vi "PH_Cam_BaseClass.get Cam Attribute.vi"(0 "IMAQ1394 Session In":T3, 1 "Cam Number Attribute Name":string, 2 "Attribute Information Array":T2(array[cluster]), 5 "error in (no error)":errorcluster) -> (6 "Current String Value":string, 7 "Attribute writable?":bool, 8 "Current Bool Value":bool, 9 "EnumValues[]":u32[](array[numeric]), 10 "Comment/Attribute Type":string, 11 "EnumStrings[]":string[](array[string]), 12 "Attribute read?":bool, 13 "Description":string, 14 "IMAQ1394 Session Out":T3, 15 "Current Num Value":dbl, 16 "Maximum":dbl, 17 "Minimum":dbl, 18 "Units":string, 19 "error out":errorcluster)   [LabVIEW 2014]
doc: "This VI gets a camera attribute."
uses:
  <vilib>/userdefined/High Color/IMAQdx.ctl
  <vilib>/vision/driver/IMAQdx.llb/IMAQdx Attribute Type.ctl
  <resource>/objmgr/imaqdx.rc
  <vilib>/vision/driver/NI_Vision_Acquisition_Software.lvlib
panel:
  in  "Attribute Type":T1
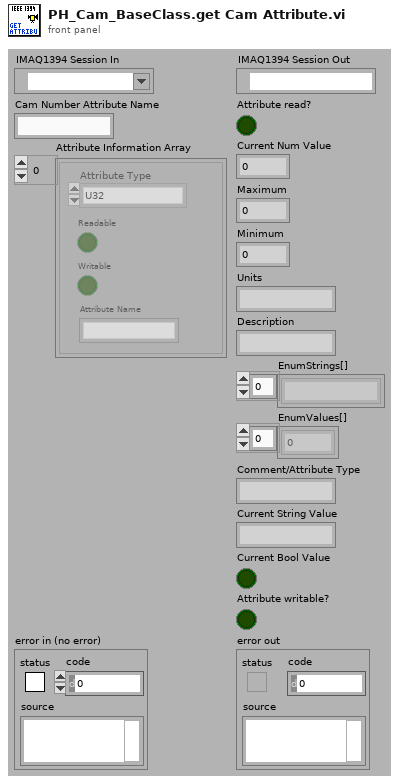
[diagram p1: front panel]
types:
  T1 = typedef "NI_Vision_Acquisition_Software.lvlib/IMAQdx Attribute Type.ctl" = enum32{"U32", "I64", "DBL", "String", "Enum", "Bool", "Command"}
  T2 = cluster{"Attribute Type":T1, "Readable":bool, "Writable":bool, "Attribute Name":string}[]
  T3 = typedef "IMAQdx.ctl" = refnum<k21>
  T4 = cluster{"Attribute Type":T1, "Readable":bool, "Writable":bool, "Attribute Name":string}
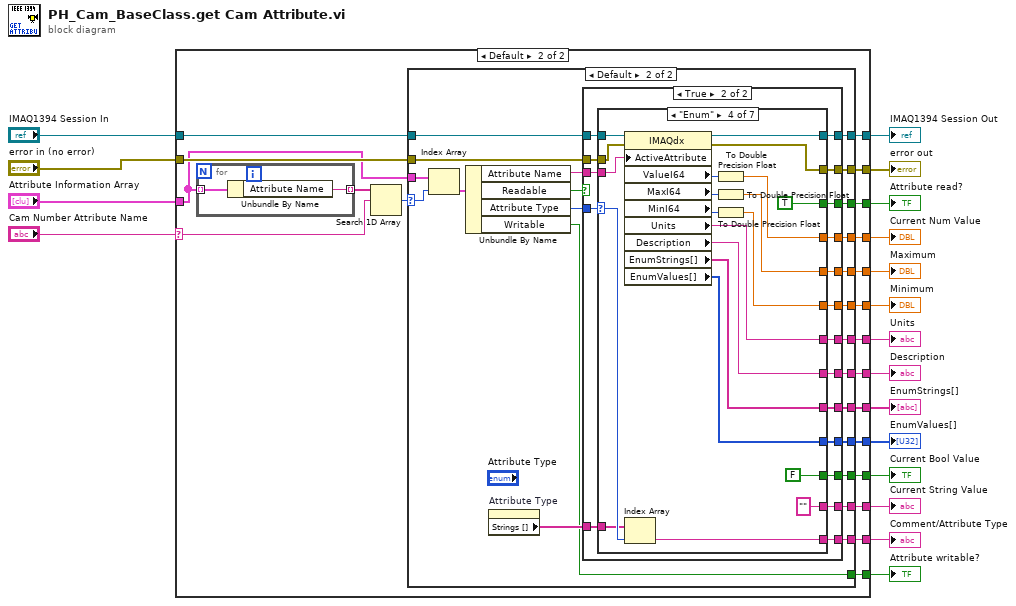
[diagram p0: block diagram]
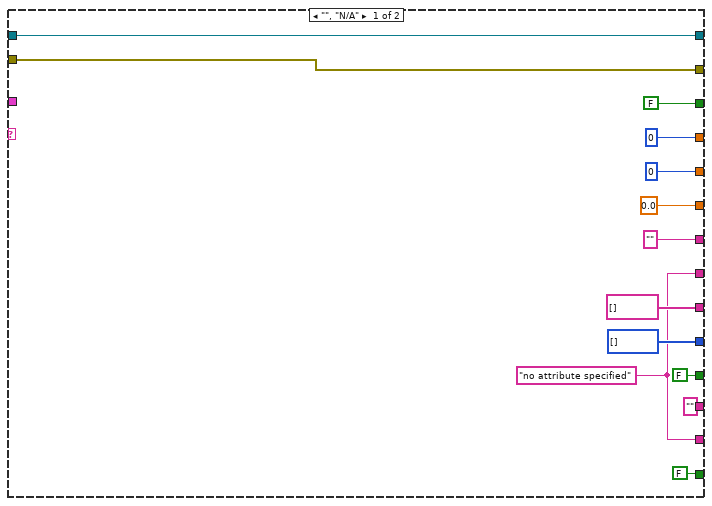
[diagram p2: hidden frame]
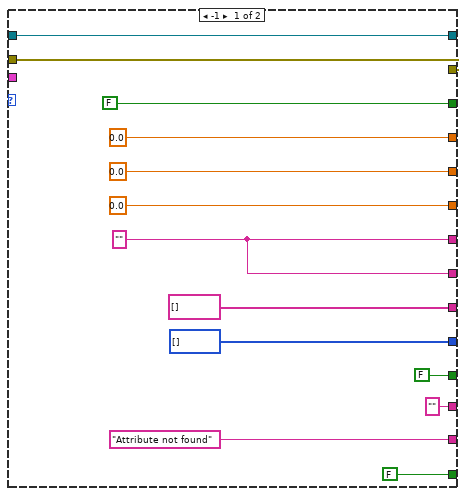
[diagram p3: hidden frame]
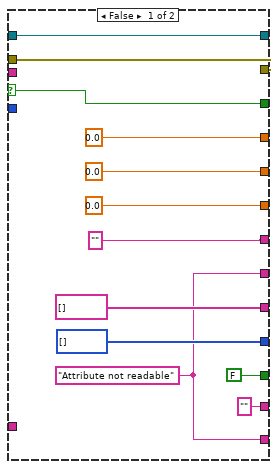
[diagram p4: hidden frame]
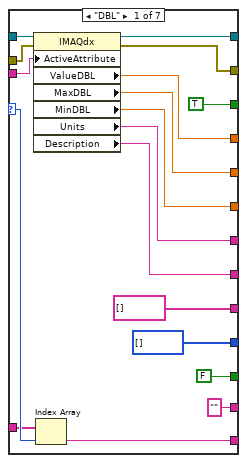
[diagram p5: hidden frame]
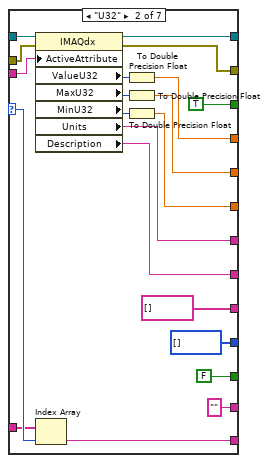
[diagram p6: hidden frame]
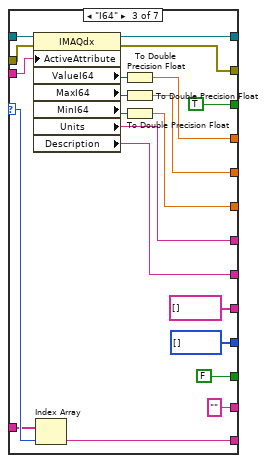
[diagram p7: hidden frame]
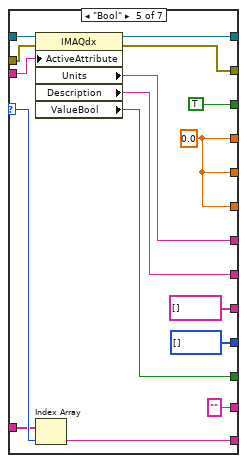
[diagram p8: hidden frame]
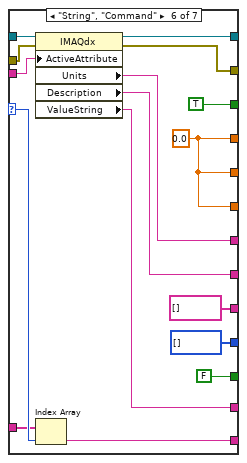
[diagram p9: hidden frame]
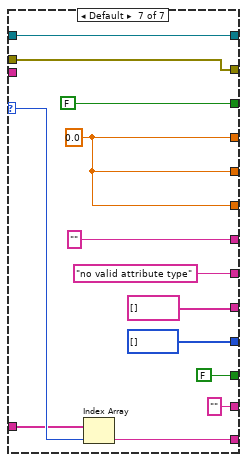
[diagram p10: hidden frame]
diagram:
  n1 = case shown="Default" "Cam Number Attribute Name" {
    selector: "Cam Number Attribute Name" -> [_ w47]
    tunnel: [w31 w51] -> w18
    tunnel: [w30 w50] -> w17
    tunnel: "error in (no error)" -> [w30 w49]
    tunnel: "IMAQ1394 Session In" -> [w31 w46]
    tunnel: [FALSE w48] -> w14
    tunnel: [u32 0 ("ValueU32") w45] -> w12
    tunnel: [w22 w44] -> w11
    tunnel: [i64 0 ("ValueI64") w43] -> w10
    tunnel: [0.0 ("ValueDBL") w42] -> w9
    tunnel: ["" ("ValueString") w41] -> w8
    tunnel: [w22 w40] -> w7
    tunnel: [string[] [] ("EnumStrings[]") w39] -> w6
    tunnel: [u32[] [] ("EnumValues[]") w38] -> w5
    tunnel: [FALSE ("Writable") w37] -> w4
    tunnel: [FALSE ("ValueBool") w36] -> w3
    tunnel: ["" ("ValueString") w35] -> w2
    tunnel: "Attribute Information Array" -> [_ w34]
    frame "", "N/A" {
      w22 = "no attribute specified"
    }
    frame Default {
      n2 = for {
        tunnel: w34 -> [w245] mode=indexing
        tunnel: [w244] -> w33 mode=indexing
        n3 = Unbundle By Name(w245) -> ("Attribute Name"=w244:string)
      }
      n4 = Search 1D Array(1D array=w33, element=w47) -> (index of element=w32:i32)  [unwired: 1 in]
      n5 = case shown="Default" w32 {
        selector: w32 -> [_ w81]
        tunnel: [w63 w87] -> w51
        tunnel: w49 -> [w64 w86]
        tunnel: [w64 w85] -> w50
        tunnel: w46 -> [w63 w84]
        tunnel: w34 -> [_ w83]
        tunnel: [FALSE w78] -> w48
        tunnel: [0.0 ("ValueU32") w76] -> w45
        tunnel: ["Attribute not found" w74] -> w44
        tunnel: [0.0 ("ValueI64") w73] -> w43
        tunnel: [0.0 ("ValueDBL") w72] -> w42
        tunnel: [w57 w71] -> w41
        tunnel: [w57 w70] -> w40
        tunnel: [string[] [] ("EnumStrings[]") w69] -> w39
        tunnel: [u32[] [] ("EnumValues[]") w68] -> w38
        tunnel: [FALSE ("Writable") w67] -> w37
        tunnel: [FALSE ("ValueBool") w66] -> w36
        tunnel: ["" ("ValueString") w65] -> w35
        frame -1 {
          w57 = "" ("ValueString")
        }
        frame Default {
          n6 = Index Array(array=w83, index=w81) -> (element=w82:T4)
          n7 = Unbundle By Name(w82) -> ("Attribute Name"=w80:string, "Readable"=w79:bool, "Attribute Type"=w77:T1, "Writable"=w67:bool)
          n8 = property on="Attribute Type" class="Enum (strict)"() -> ("Strings []"=w75:string[])  [unwired: 2 in, 2 out]
          n9 = case shown="True" w79 {
            selector: w79 -> [w97 _]
            tunnel: [w99 w117] -> w87
            tunnel: w86 -> [w98 w116]
            tunnel: [w98 w115] -> w85
            tunnel: w84 -> [w99 w114]
            tunnel: w80 -> [_ w113]
            tunnel: [w97 w112] -> w78
            tunnel: w77 -> [_ w107]
            tunnel: [0.0 ("ValueU32") w111] -> w76
            tunnel: w75 -> [_ w106]
            tunnel: [w90 w105] -> w74
            tunnel: [0.0 ("ValueI64") w110] -> w73
            tunnel: [0.0 ("ValueDBL") w109] -> w72
            tunnel: ["" ("ValueString") w108] -> w71
            tunnel: [w90 w104] -> w70
            tunnel: [string[] [] ("EnumStrings[]") w103] -> w69
            tunnel: [u32[] [] ("EnumValues[]") w102] -> w68
            tunnel: [FALSE ("ValueBool") w101] -> w66
            tunnel: ["" ("ValueString") w100] -> w65
            frame False {
              w90 = "Attribute not readable"
            }
            frame True {
              n10 = case shown="\"Enum\"" w107 {
                selector: w107 -> [w129 w150 w171 w192 w208 w224 w242]
                tunnel: [w135 w156 w177 w198 w214 w230 w239] -> w117
                tunnel: w116 -> [w131 w152 w173 w194 w210 w226 w238]
                tunnel: [w134 w155 w176 w197 w213 w229 w238] -> w115
                tunnel: w114 -> [w132 w153 w174 w195 w211 w227 w239]
                tunnel: w113 -> [w133 w154 w175 w196 w212 w228 _]
                tunnel: [TRUE TRUE TRUE TRUE TRUE TRUE FALSE] -> w112
                tunnel: [w124 w142 w163 w182 w199 w215 w237] -> w111
                tunnel: [w122 w141 w162 w181 w199 w215 w237] -> w110
                tunnel: [w123 w140 w161 w180 w199 w215 w237] -> w109
                tunnel: [w126 w147 w168 w189 w205 w221 "" ("Units")] -> w108
                tunnel: w106 -> [w128 w149 w170 w191 w207 w223 w241]
                tunnel: [w127 w148 w169 w190 w206 w222 w240] -> w105
                tunnel: [w125 w146 w167 w188 w204 w220 "no valid attribute type" ("Description")] -> w104
                tunnel: [string[] [] ("EnumStrings[] 2") string[] [] ("EnumStrings[] 2") string[] [] ("EnumStrings[] 2") w184 string[] [] ("EnumStrings[] 2") string[] [] ("EnumStrings[] 2") string[] [] ("EnumStrings[] 2")] -> w103
                tunnel: [u32[] [] ("EnumValues[]") u32[] [] ("EnumValues[]") u32[] [] ("EnumValues[]") w183 u32[] [] ("EnumValues[]") u32[] [] ("EnumValues[]") u32[] [] ("EnumValues[]")] -> w102
                tunnel: [FALSE ("ValueBool") FALSE ("ValueBool") FALSE ("ValueBool") FALSE ("ValueBool") w203 FALSE ("ValueBool") FALSE ("ValueBool")] -> w101
                tunnel: ["" ("ValueString") "" ("ValueString") "" ("ValueString") "" ("ValueString") "" ("ValueString") w217 "" ("ValueString")] -> w100
                frame "DBL" {
                  n11 = property class="IMAQdx"(reference=w132, error in=w131, "ActiveAttribute"=w133) -> (reference out=w135:T3, error out=w134:errorcluster, "ValueDBL"=w124:dbl, "MaxDBL"=w122:dbl, "MinDBL"=w123:dbl, "Units"=w126:string, "Description"=w125:string)
                  n12 = Index Array(array=w128, index=w129) -> (element=w127:string)
                }
                frame "U32" {
                  n13 = property class="IMAQdx"(reference=w153, error in=w152, "ActiveAttribute"=w154) -> (reference out=w156:T3, error out=w155:errorcluster, "ValueU32"=w145:u32, "MaxU32"=w143:u32, "MinU32"=w144:u32, "Units"=w147:string, "Description"=w146:string)
                  n14 = Index Array(array=w149, index=w150) -> (element=w148:string)
                  n15 = To Double Precision Float(number=w145) -> (double precision float=w142:dbl)
                  n16 = To Double Precision Float(number=w143) -> (double precision float=w141:dbl)
                  n17 = To Double Precision Float(number=w144) -> (double precision float=w140:dbl)
                }
                frame "I64" {
                  n18 = property class="IMAQdx"(reference=w174, error in=w173, "ActiveAttribute"=w175) -> (reference out=w177:T3, error out=w176:errorcluster, "ValueI64"=w166:i64, "MaxI64"=w164:i64, "MinI64"=w165:i64, "Units"=w168:string, "Description"=w167:string)
                  n19 = Index Array(array=w170, index=w171) -> (element=w169:string)
                  n20 = To Double Precision Float(number=w166) -> (double precision float=w163:dbl)
                  n21 = To Double Precision Float(number=w164) -> (double precision float=w162:dbl)
                  n22 = To Double Precision Float(number=w165) -> (double precision float=w161:dbl)
                }
                frame "Enum" {
                  n23 = property class="IMAQdx"(reference=w195, error in=w194, "ActiveAttribute"=w196) -> (reference out=w198:T3, error out=w197:errorcluster, "ValueI64"=w187:i64, "MaxI64"=w185:i64, "MinI64"=w186:i64, "Units"=w189:string, "Description"=w188:string, "EnumStrings[]"=w184:string[], "EnumValues[]"=w183:u32[])
                  n24 = Index Array(array=w191, index=w192) -> (element=w190:string)
                  n25 = To Double Precision Float(number=w187) -> (double precision float=w182:dbl)
                  n26 = To Double Precision Float(number=w185) -> (double precision float=w181:dbl)
                  n27 = To Double Precision Float(number=w186) -> (double precision float=w180:dbl)
                }
                frame "Bool" {
                  w199 = 0.0 ("ValueDBL")
                  n28 = property class="IMAQdx"(reference=w211, error in=w210, "ActiveAttribute"=w212) -> (reference out=w214:T3, error out=w213:errorcluster, "Units"=w205:string, "Description"=w204:string, "ValueBool"=w203:bool)
                  n29 = Index Array(array=w207, index=w208) -> (element=w206:string)
                }
                frame "String", "Command" {
                  w215 = 0.0 ("ValueDBL")
                  n30 = property class="IMAQdx"(reference=w227, error in=w226, "ActiveAttribute"=w228) -> (reference out=w230:T3, error out=w229:errorcluster, "Units"=w221:string, "Description"=w220:string, "ValueString"=w217:string)
                  n31 = Index Array(array=w223, index=w224) -> (element=w222:string)
                }
                frame Default {
                  w237 = 0.0 ("ValueDBL")
                  n32 = Index Array(array=w241, index=w242) -> (element=w240:string)
                }
              }
            }
          }
        }
      }
    }
  }
  "error out" <- w17
  "Attribute read?" <- w14
  "IMAQ1394 Session Out" <- w18
  "Current Num Value" <- w12
  "Comment/Attribute Type" <- w11
  "Maximum" <- w10
  "Minimum" <- w9
  "Units" <- w8
  "Description" <- w7
  "EnumStrings[]" <- w6
  "EnumValues[]" <- w5
  "Attribute writable?" <- w4
  "Current Bool Value" <- w3
  "Current String Value" <- w2
